vi "DashboardInterface.vi"   [LabVIEW 2014]
uses:
  Robot Global Data.vi
  <vilib>/Rock Robotics/Network Tables/SD Write Number.vi
types:
  T1 = typedef "WPI_DriverStationRobotMode2.ctl" = enum16{"Autonomous Disabled", "Autonomous Enabled", "Teleop Disabled", "Teleop Enabled", "Disconnected", "Finish", "Test Disabled", "Test Enabled", "Emergency Stopped"}
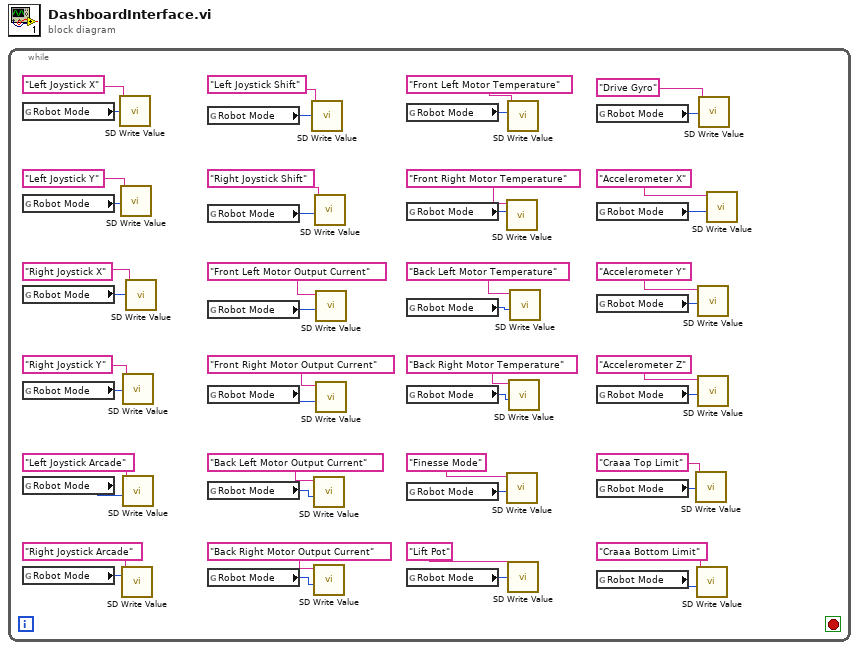
[diagram p0: block diagram]
diagram:
  n1 = while {
    stop <- _ stop-if-true
    n2 = global read "Robot Global Data.vi" "Robot Mode"() -> (w45:T1)
    n3 = global read "Robot Global Data.vi" "Robot Mode"() -> (w47:T1)
    n4 = global read "Robot Global Data.vi" "Robot Mode"() -> (w43:T1)
    n5 = global read "Robot Global Data.vi" "Robot Mode"() -> (w41:T1)
    n6 = global read "Robot Global Data.vi" "Robot Mode"() -> (w39:T1)
    n7 = global read "Robot Global Data.vi" "Robot Mode"() -> (w37:T1)
    n8 = call-poly <vilib>:"SD Write Value.vi"("Numeric"=w45, "Name"="Left Joystick X") -> ()  [unwired: 8 in, 2 out]
    n9 = call-poly <vilib>:"SD Write Value.vi"("Numeric"=w47, "Name"="Left Joystick Y") -> ()  [unwired: 8 in, 2 out]
    n10 = call-poly <vilib>:"SD Write Value.vi"("Numeric"=w37, "Name"="Right Joystick Arcade") -> ()  [unwired: 8 in, 2 out]
    n11 = call-poly <vilib>:"SD Write Value.vi"("Numeric"=w41, "Name"="Right Joystick Y") -> ()  [unwired: 8 in, 2 out]
    n12 = call-poly <vilib>:"SD Write Value.vi"("Numeric"=w39, "Name"="Left Joystick Arcade") -> ()  [unwired: 8 in, 2 out]
    n13 = call-poly <vilib>:"SD Write Value.vi"("Numeric"=w43, "Name"="Right Joystick X") -> ()  [unwired: 8 in, 2 out]
    n14 = global read "Robot Global Data.vi" "Robot Mode"() -> (w35:T1)
    n15 = global read "Robot Global Data.vi" "Robot Mode"() -> (w33:T1)
    n16 = global read "Robot Global Data.vi" "Robot Mode"() -> (w31:T1)
    n17 = global read "Robot Global Data.vi" "Robot Mode"() -> (w29:T1)
    n18 = global read "Robot Global Data.vi" "Robot Mode"() -> (w27:T1)
    n19 = global read "Robot Global Data.vi" "Robot Mode"() -> (w25:T1)
    n20 = call-poly <vilib>:"SD Write Value.vi"("Numeric"=w35, "Name"="Left Joystick Shift") -> ()  [unwired: 8 in, 2 out]
    n21 = call-poly <vilib>:"SD Write Value.vi"("Numeric"=w27, "Name"="Back Left Motor Output Current") -> ()  [unwired: 8 in, 2 out]
    n22 = call-poly <vilib>:"SD Write Value.vi"("Numeric"=w25, "Name"="Back Right Motor Output Current") -> ()  [unwired: 8 in, 2 out]
    n23 = call-poly <vilib>:"SD Write Value.vi"("Numeric"=w33, "Name"="Right Joystick Shift") -> ()  [unwired: 8 in, 2 out]
    n24 = call-poly <vilib>:"SD Write Value.vi"("Numeric"=w31, "Name"="Front Left Motor Output Current") -> ()  [unwired: 8 in, 2 out]
    n25 = call-poly <vilib>:"SD Write Value.vi"("Numeric"=w29, "Name"="Front Right Motor Output Current") -> ()  [unwired: 8 in, 2 out]
    n26 = global read "Robot Global Data.vi" "Robot Mode"() -> (w23:T1)
    n27 = global read "Robot Global Data.vi" "Robot Mode"() -> (w21:T1)
    n28 = global read "Robot Global Data.vi" "Robot Mode"() -> (w19:T1)
    n29 = global read "Robot Global Data.vi" "Robot Mode"() -> (w17:T1)
    n30 = global read "Robot Global Data.vi" "Robot Mode"() -> (w15:T1)
    n31 = global read "Robot Global Data.vi" "Robot Mode"() -> (w13:T1)
    n32 = call-poly <vilib>:"SD Write Value.vi"("Numeric"=w21, "Name"="Front Right Motor Temperature") -> ()  [unwired: 8 in, 2 out]
    n33 = call-poly <vilib>:"SD Write Value.vi"("Numeric"=w15, "Name"="Finesse Mode") -> ()  [unwired: 8 in, 2 out]
    n34 = call-poly <vilib>:"SD Write Value.vi"("Numeric"=w23, "Name"="Front Left Motor Temperature") -> ()  [unwired: 8 in, 2 out]
    n35 = call-poly <vilib>:"SD Write Value.vi"("Numeric"=w13, "Name"="Lift Pot") -> ()  [unwired: 8 in, 2 out]
    n36 = call-poly <vilib>:"SD Write Value.vi"("Numeric"=w17, "Name"="Back Right Motor Temperature") -> ()  [unwired: 8 in, 2 out]
    n37 = call-poly <vilib>:"SD Write Value.vi"("Numeric"=w19, "Name"="Back Left Motor Temperature") -> ()  [unwired: 8 in, 2 out]
    n38 = global read "Robot Global Data.vi" "Robot Mode"() -> (w11:T1)
    n39 = global read "Robot Global Data.vi" "Robot Mode"() -> (w9:T1)
    n40 = global read "Robot Global Data.vi" "Robot Mode"() -> (w7:T1)
    n41 = global read "Robot Global Data.vi" "Robot Mode"() -> (w5:T1)
    n42 = global read "Robot Global Data.vi" "Robot Mode"() -> (w3:T1)
    n43 = global read "Robot Global Data.vi" "Robot Mode"() -> (w1:T1)
    n44 = call-poly <vilib>:"SD Write Value.vi"("Numeric"=w3, "Name"="Craaa Top Limit") -> ()  [unwired: 8 in, 2 out]
    n45 = call-poly <vilib>:"SD Write Value.vi"("Numeric"=w1, "Name"="Craaa Bottom Limit") -> ()  [unwired: 8 in, 2 out]
    n46 = call-poly <vilib>:"SD Write Value.vi"("Numeric"=w7, "Name"="Accelerometer Y") -> ()  [unwired: 8 in, 2 out]
    n47 = call-poly <vilib>:"SD Write Value.vi"("Numeric"=w5, "Name"="Accelerometer Z") -> ()  [unwired: 8 in, 2 out]
    n48 = call-poly <vilib>:"SD Write Value.vi"("Numeric"=w11, "Name"="Drive Gyro") -> ()  [unwired: 8 in, 2 out]
    n49 = call-poly <vilib>:"SD Write Value.vi"("Numeric"=w9, "Name"="Accelerometer X") -> ()  [unwired: 8 in, 2 out]
  }
